vi "avarage_images.vi"(8 "error in (no error)":errorcluster, 9 "Exposure Time (s)":dbl=0.004 min=0.0 step=0.001 format="%.3f", 10 "Number of Images":u32=1 min=1 step=1, 11 "Camera Handle":u32) -> (0 "error out":errorcluster, 1 "Image Avarage":dbl[](array[numeric]), 2 "Number of Images":u32=1 min=1 step=1, 3 "Camera Handle":u32, 5 "Waveform Graph":i32[](graph))   [LabVIEW 2014]
panel:
  out "PyLoN Ready":bool
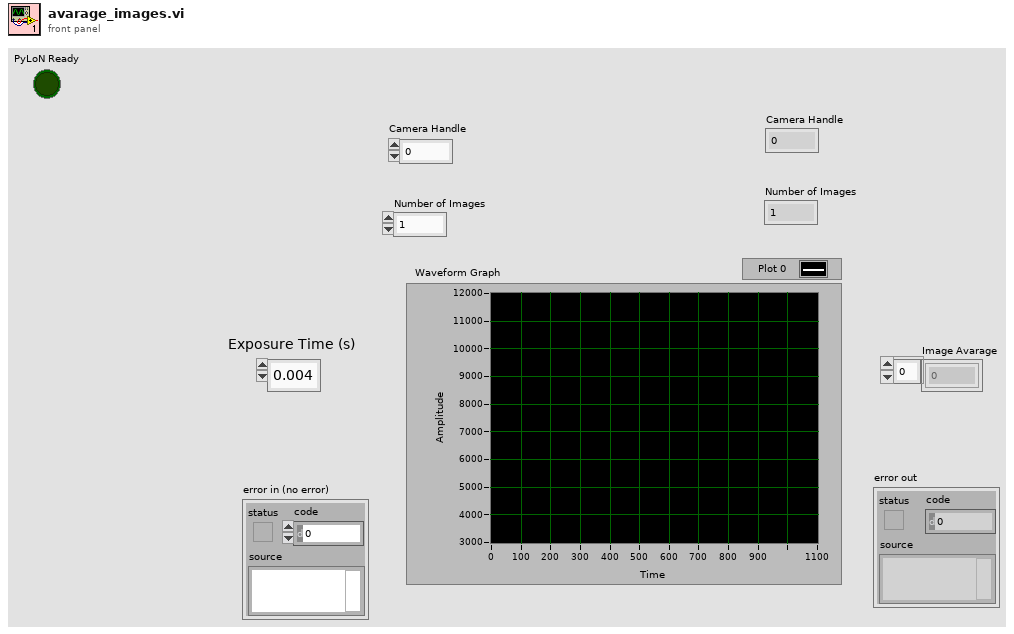
[diagram p1: front panel]
types:
  T1 = cluster{"acquire focus mode":u32, "Exposure Time (s)":dbl, i32, "Software accumulation":u32}
  T2 = cluster{"Camera Handle":u32, "Pulser Handle":u32, "File Handle":u32, "Display Handle":u32, "Image Handle":u32}
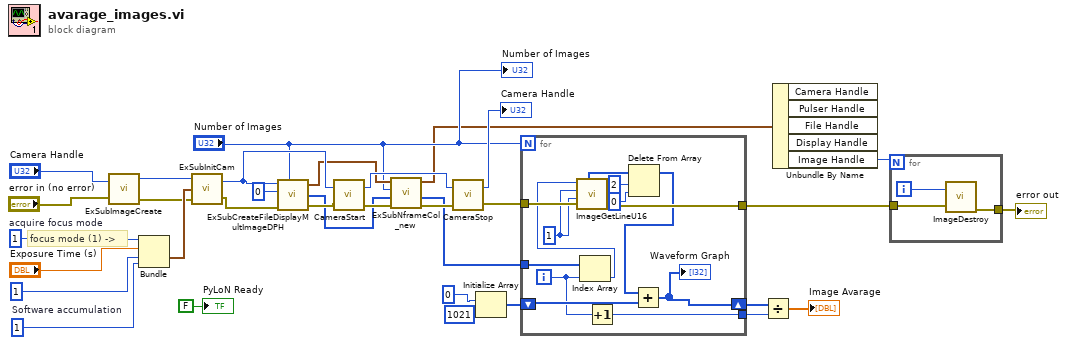
[diagram p0: block diagram]
diagram:
  w32 = u32 1  # acquire focus mode
  w31 = u32 1  # Software accumulation
  # "focus mode (1) ->"
  n1 = call "ExSubImageCreate.vi"("Camera Handle"="Camera Handle", "error in (no error)"="error in (no error)") -> ("Camera Handle"=w30:u32, "error out"=w29:errorcluster)  [unwired: 1 out]
  n2 = Bundle("acquire focus mode"=w32, "Exposure Time (s)"="Exposure Time (s)", 1, "Software accumulation"=w31) -> (w33:T1)  [unwired: 1 in]
  n3 = call "ExSubInitCam.vi"("error in (no error)"=w29, "Camera Information"=w33, "Camera Handle"=w30) -> ("error out"=w14:errorcluster, "Camera Handle"=w12:u32)
  n4 = call "ExSubCreateFileDisplayMultImageDPH.vi"("Camera Handle"=w12, "Pulser Handle"=u32 0, "error in (no error)"=w14, "Number of Images"="Number of Images") -> ("Handles Out"=w6:T2, "Array"=w4:u32[], "error out"=w13:errorcluster)  [unwired: 1 in]
  n5 = call <userlib>:"CameraStart.vi"("error in"=w13, "Camera Handle"=w12) -> ("error out"=w7:errorcluster, "Camera Handle"=w23:u32)
  n6 = call "ExSubNframeCol_new.vi"("error in (no error)"=w7, "image handles"=w4, "Number of Images"="Number of Images", "Handle Cluster 2"=w6) -> ("error out"=w3:errorcluster, "data handles"=w2:u32[], "Handle Cluster"=w1:T2)  [unwired: 4 in, 1 out]
  n7 = call <userlib>:"CameraStop.vi"("error in"=w3, "Camera Handle"=w23) -> ("error out"=w24:errorcluster, "Camera Handle"=→"Camera Handle":u32)
  n8 = Initialize Array(0, 1021 ("dimension size")) -> (w8:i32[])
  n9 = for {
    N: "Number of Images" -> [_]
    tunnel: w2 -> [w46]
    tunnel: w24 -> [w45]
    tunnel: [w35] -> w20
    shift-right: [w41] -> w17
    shift-left: w8 -> [w42]
    tunnel: [w39] -> w16
    i -> [w40]
    w44 = u32 1
    n10 = Index Array(array=w46, index=w40) -> (element=w43:u32)
    n11 = call <userlib>:"ImageGetLineU16.vi"("Data Handle"=w43, "Y Position"=w44, "Z Position"=w44, "error in"=w45) -> ("Array u16"=w38:u16[], "error out"=w35:errorcluster)  [unwired: 1 out]
    n12 = Increment(x=w40) -> (x+1=w39:i32)
    n13 = Delete From Array(array=w38, length=2, index=0) -> (array with subset deleted=w34:u16[])  [unwired: 1 out]
    n14 = Add(x=w34, y=w42) -> (x+y=w41:i32[])
    "Waveform Graph" <- w41
  }
  n15 = Divide(x=w17, y=w16) -> (x/y=→"Image Avarage":dbl[])
  n16 = Unbundle By Name(w1) -> ("Image Handle"=w21:u32)  [unwired: 4 out]
  n17 = for {
    N: w21 -> [_]
    tunnel: [w49] -> w22
    tunnel: w20 -> [w48]
    i -> [w47]
    n18 = call <userlib>:"ImageDestroy.vi"("error in"=w48, "Data handle"=w47) -> ("error out"=w49:errorcluster)
  }
  "error out" <- w22
  "PyLoN Ready" <- FALSE ("PyLoN Ready")
  "Number of Images" <- "Number of Images"
